vi "Additional.vi"() -> ()   [LabVIEW 2017]
panel:
  out "appended array":dbl[](array[numeric])
  in  "stop 2":bool
  out "Waveform Chart 2":waveform(dbl)(graph)
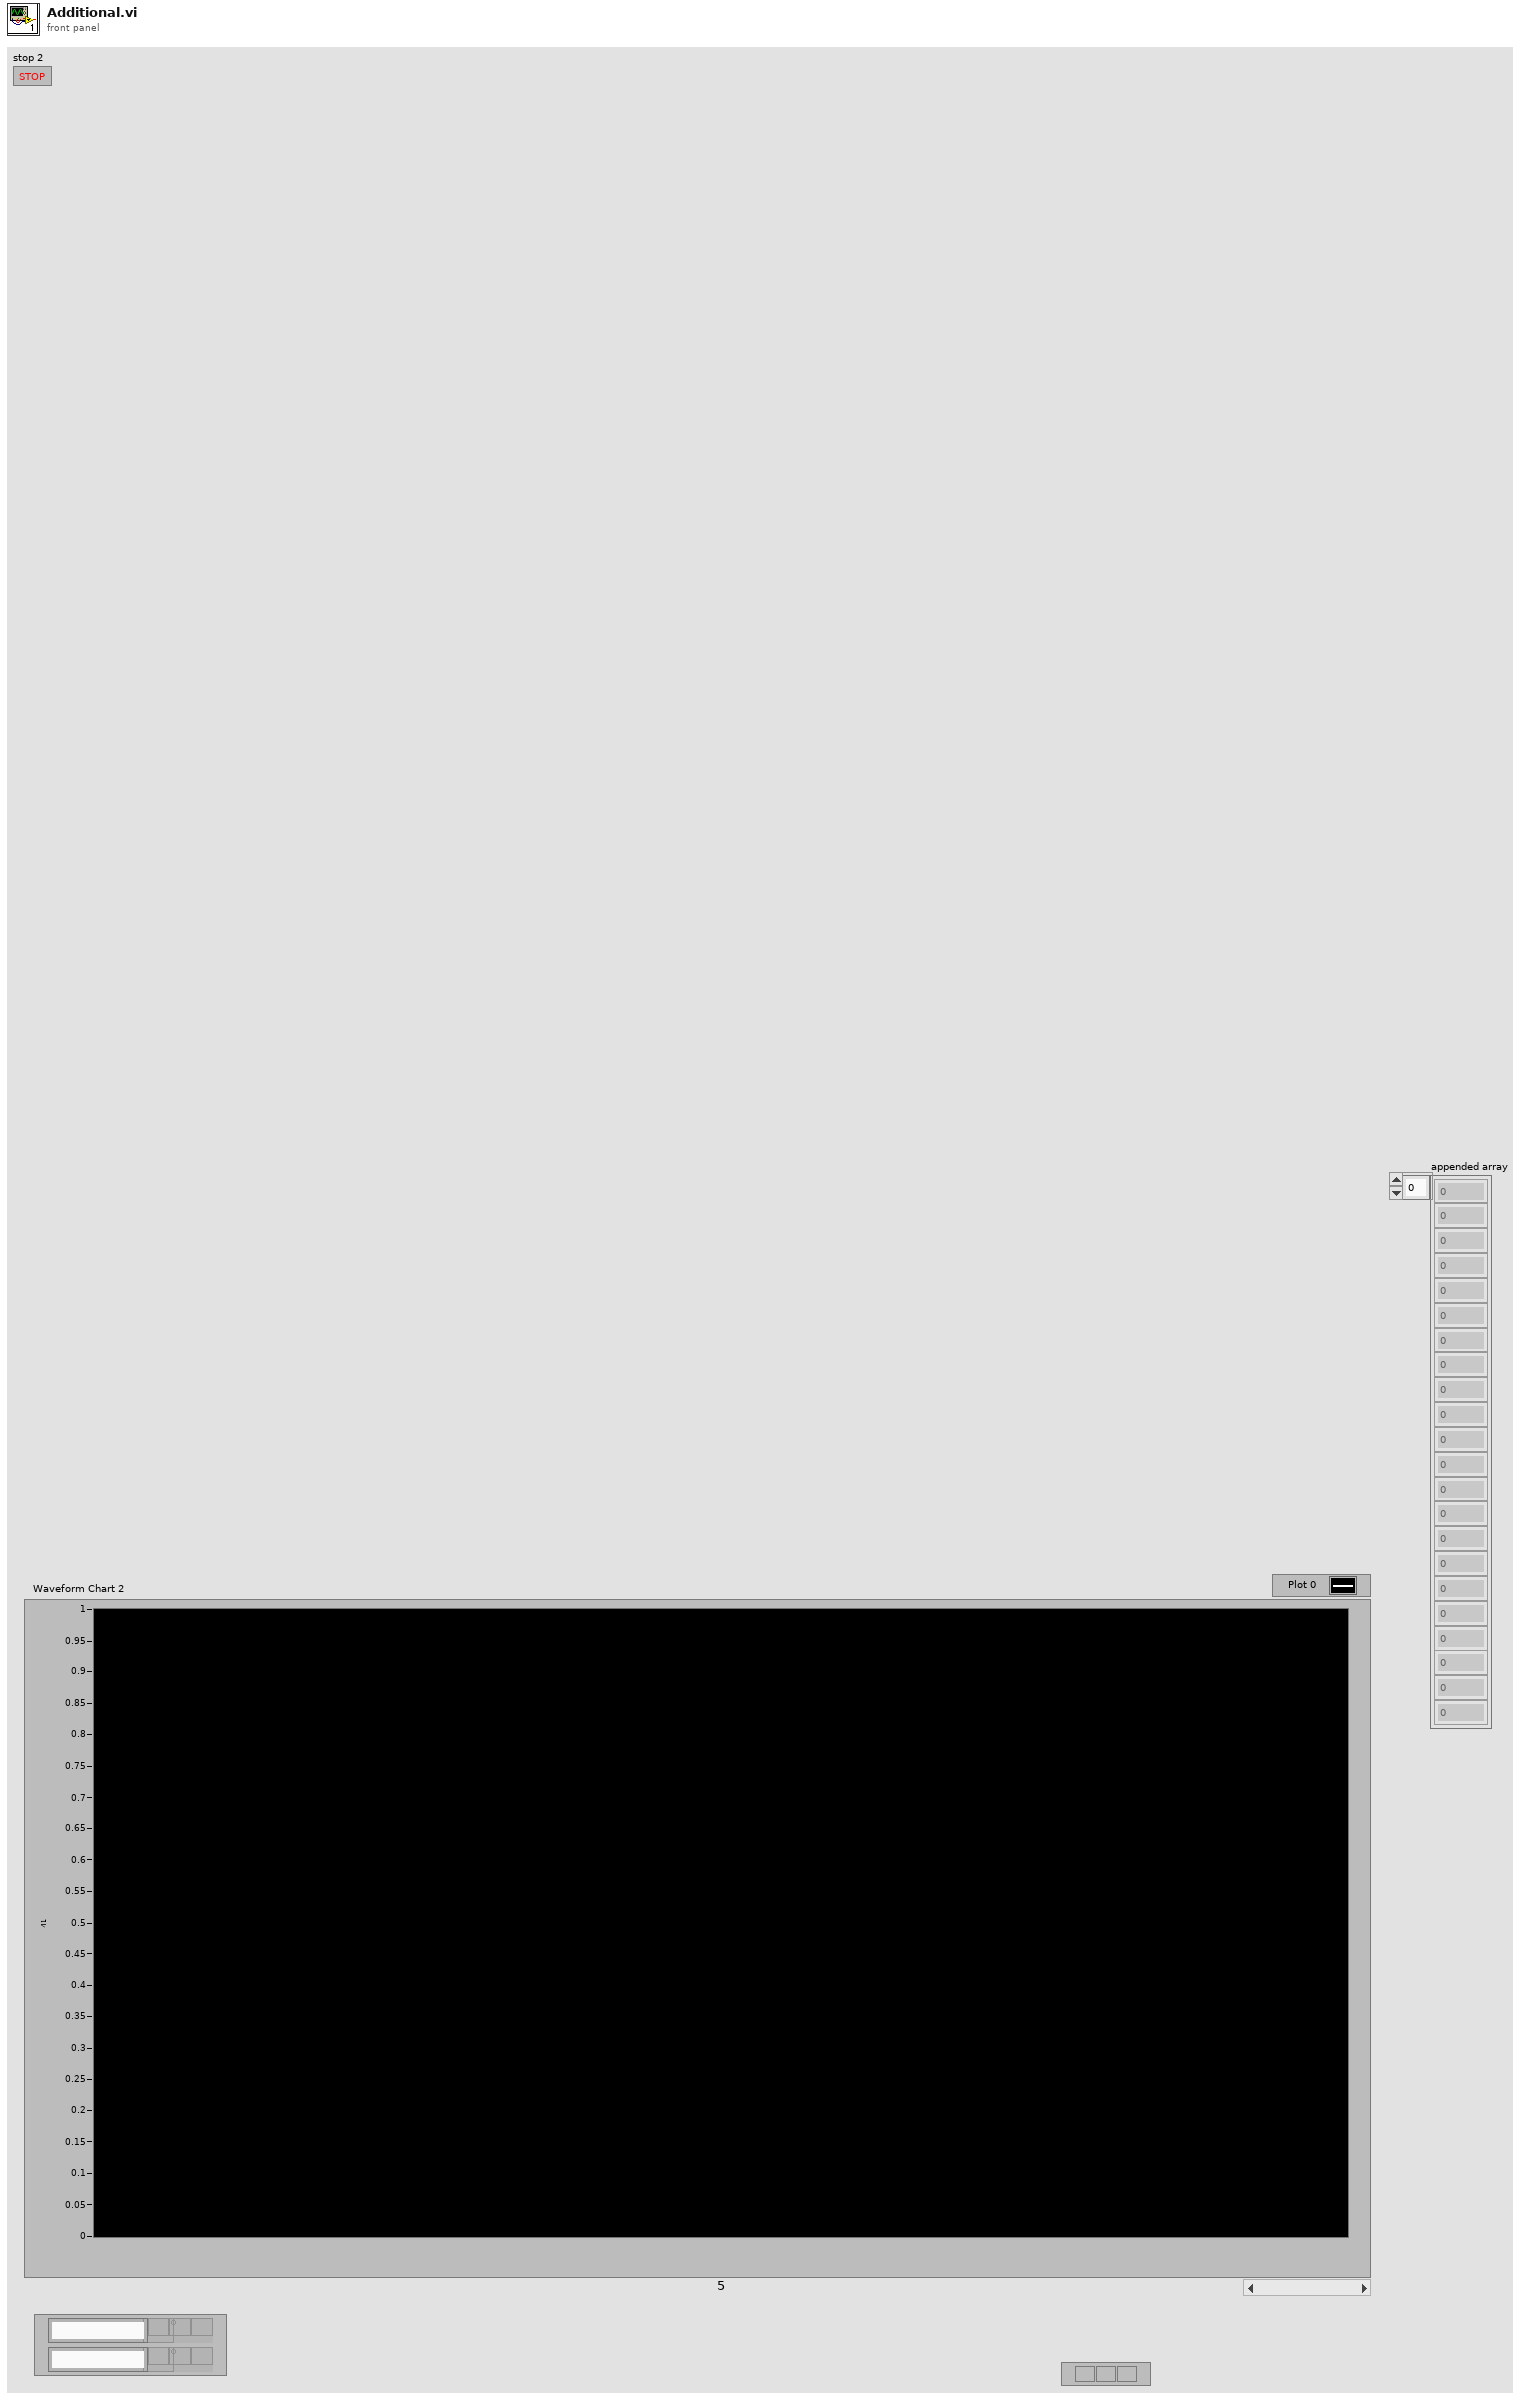
[diagram p1: front panel]
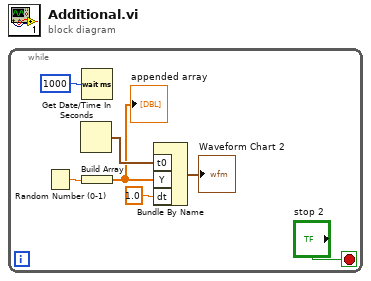
[diagram p0: block diagram]
diagram:
  n1 = while {
    stop <- "stop 2" stop-if-true
    n2 = Random Number (0-1)() -> (number: 0 to 1=w5:dbl)
    n3 = Get Date/Time In Seconds() -> (seconds since 1Jan1904=w7:timestamp)
    n4 = Wait (ms)(milliseconds to wait=u32 1000 ("millisecond multiple")) -> ()  [unwired: 1 out]
    n5 = Build Array(w5) -> (w6:dbl[])
    "appended array" <- w6
    n6 = Bundle By Name("t0"=w7, "Y"=w6, "dt"=1.0) -> (→"Waveform Chart 2":waveform(dbl))  [unwired: 1 in]
  }
